vi "CreatePipeSeparatedList.vi"(10 "Array":string[](array[string]), 11 "List In":string) -> (3 "List Out":string)   [LabVIEW 2017]
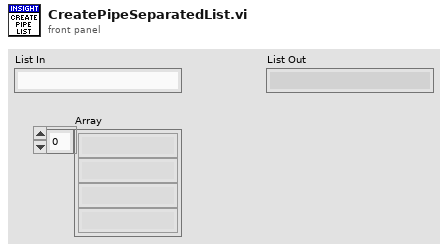
[diagram p1: front panel]
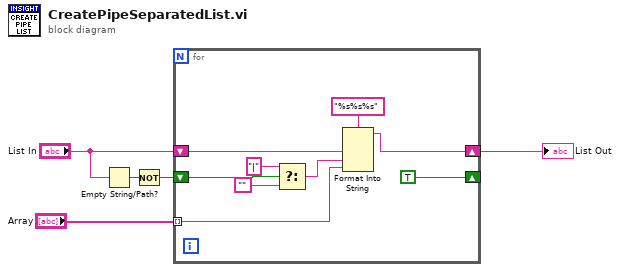
[diagram p0: block diagram]
diagram:
  n1 = Empty String/Path?(string/path="List In") -> (empty?=w5:bool)
  n2 = Not(x=w5) -> (.not. x?=w4:bool)
  n3 = for {
    tunnel: "Array" -> [w10] mode=indexing
    shift-right: [w11] -> w3
    shift-left: "List In" -> [w13]
    shift-right: [TRUE] -> _
    shift-left: w4 -> [w14]
    n4 = Select(t="|", s=w14, f="") -> (s? t:f=w6:string)
    n5 = Format Into String(format string="%s%s%s", w13, w6, w10) -> (resulting string=w11:string)  [unwired: 2 in, 1 out]
  }
  "List Out" <- w3
